vi "read from binary file.vi"() -> ()   [LabVIEW 2016]
panel:
  out "Waveform Graph":dbl[](graph)
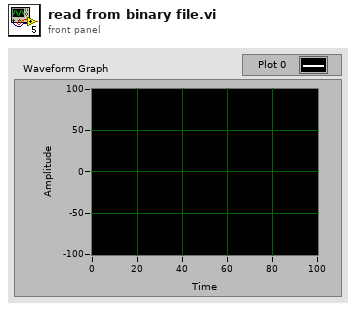
[diagram p1: front panel]
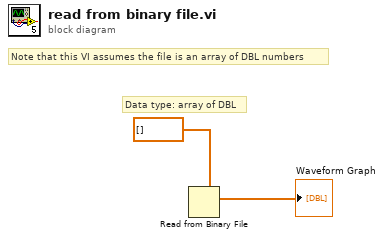
[diagram p0: block diagram]
diagram:
  # "Note that this VI assumes the file is an array of DBL numbers"
  # "Data type: array of DBL"
  n1 = Read from Binary File(5:dbl[] []) -> (2:→"Waveform Graph":dbl[])  [unwired: 5 in, 3 out]
